vi "Banda_HMI_UART.vi"() -> ()   [LabVIEW 2026]
uses:
  <vilib>/Instr/_visa.llb/VISA Configure Serial Port (Instr).vi
panel:
  in  "VELOCIDAD BANDA":u8(knob) scale=0.0..100.0 scale format="%^#.6g"
  in  "BRAZO CLASIFICADOR":bool
  in  "MOTOR BANDA":bool
  out "Trama":bool
  in  "stop":bool
  out "CONTADOR PIEZAS":u16
  out "SENSOR DE PRESENCIA":bool
  out "TEMPERATURA":u8(slide) scale=0.0..100.0
  out "SOBRECALENTAMIENTO":bool
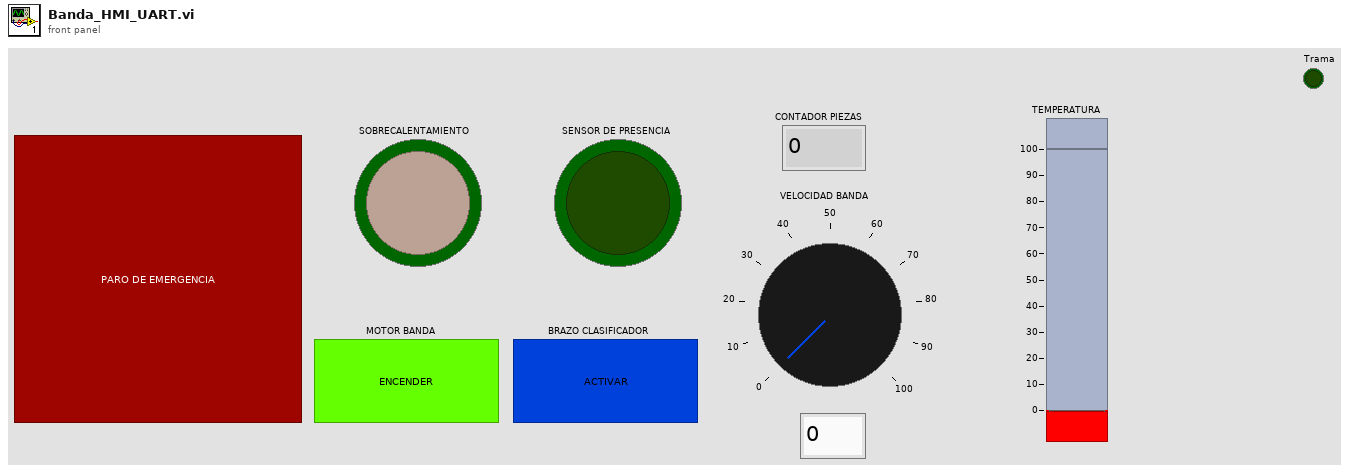
[diagram p1: front panel]
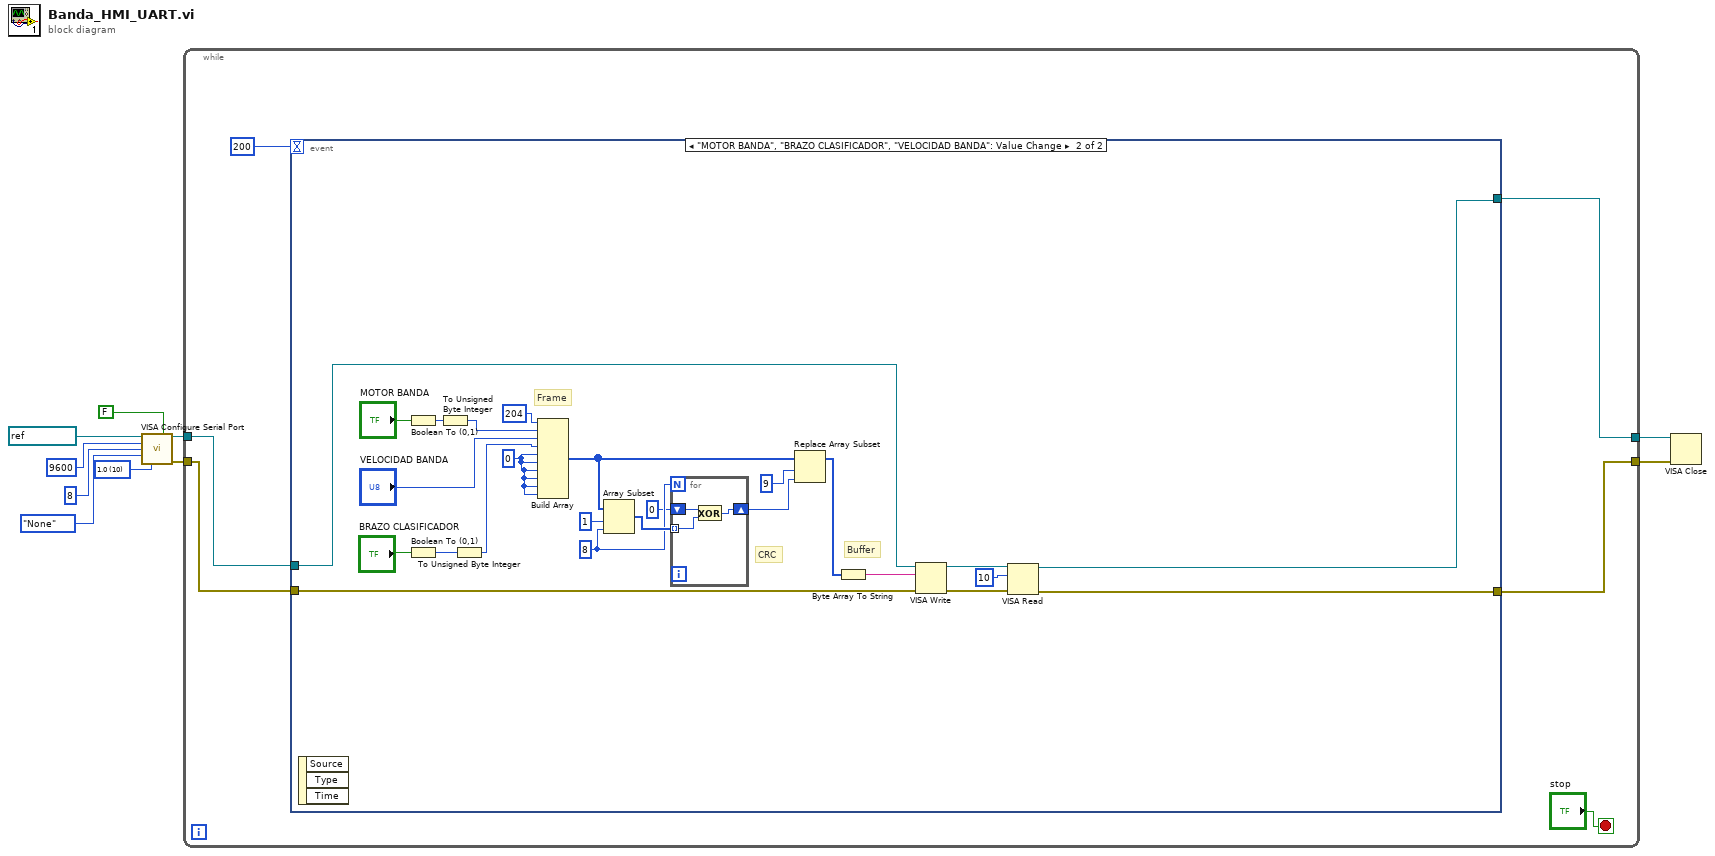
[diagram p0: block diagram]
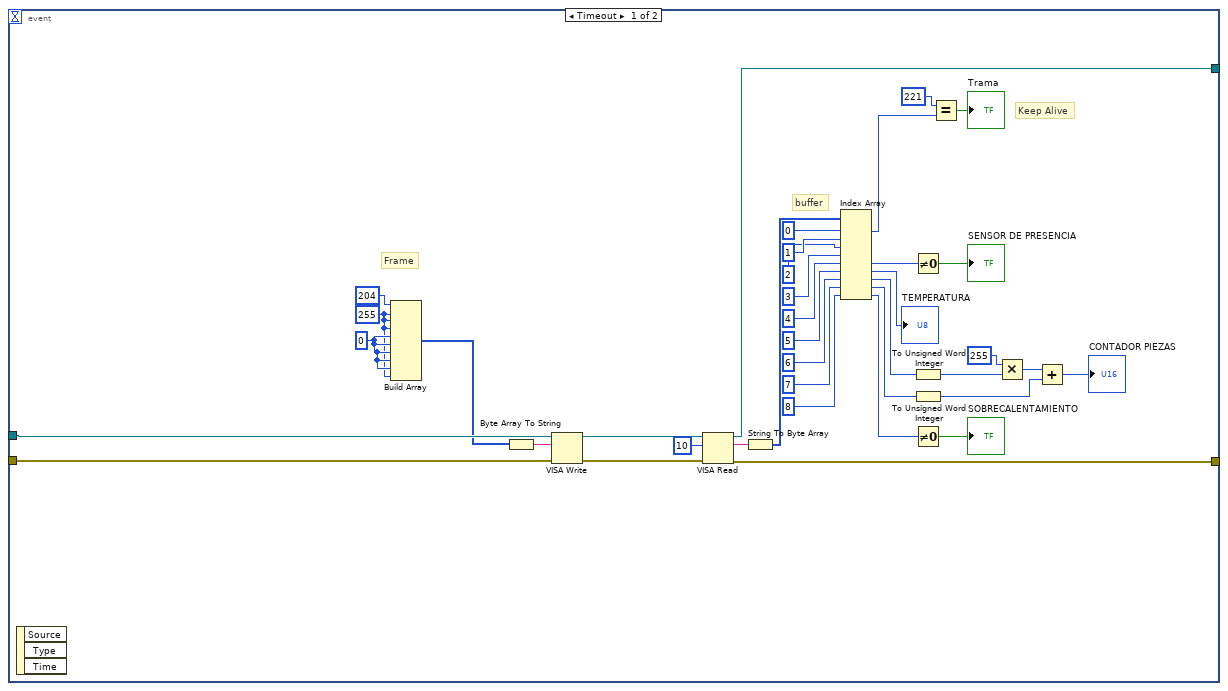
[diagram p2: hidden frame]
diagram:
  w6 = u16 10 items=["1.0"=10, "1.5"=15, "2.0"=20] ("stop bits (10: 1 bit)")
  n1 = call-poly "VISA Configure Serial Port"("VISA resource name"=refnum<visa-resource-name> "COM15", "Enable Termination\nChar (T)"=FALSE ("Enable Termination\nChar (T)"), "baud rate (9600)"=u32 9600, "data bits (8)"=u16 8, "parity (0:none)"=enum16{"None", "Odd", "Even", "Mark", "Space"}."None", "stop bits (10: 1 bit)"=w6) -> ("VISA resource name out"=w3:refnum<visa-resource-name>, "error out"=w2:errorcluster)  [unwired: 8 in]
  n2 = while {
    tunnel: w3 -> [w15]
    tunnel: [w12] -> w4
    tunnel: w2 -> [w14]
    tunnel: [w11] -> w1
    stop <- "stop" stop-if-true
    n3 = event shown="[1] \"MOTOR BANDA\", \"BRAZO CLASIFICADOR\", \"VELOCIDAD BANDA\": Value Change" {
      selector: _ -> [_ _]
      dyn-events: _ -> [_ _]
      timeout: 200 -> [_ _]
      tunnel: w15 -> [w19 w62]
      tunnel: w14 -> [w20 w61]
      tunnel: [w24 w57] -> w11
      tunnel: [w23 w58] -> w12
      event Timeout {
        w17 = u8 255 ("element")
        w52 = u8 0 ("element")
        # "Keep Alive"
        # "buffer"
        # "Frame"
        n4 = event-data() -> ()  [unwired: 1 in, 3 out]
        n5 = Build Array(u8 204 ("element"), w17, w17, w17, w52, w52, w52, w52, w52, w17) -> (w18:u8[])
        n6 = Byte Array To String(unsigned byte array=w18) -> (string=w54:string)
        n7 = VISA Write(VISA resource name=w19, write buffer=w54, error in (no error)=w20) -> (VISA resource name out=w21:refnum<visa-resource-name>, error out=w22:errorcluster)  [unwired: 1 out]
        n8 = VISA Read(VISA resource name=w21, byte count=u32 10, error in (no error)=w22) -> (VISA resource name out=w23:refnum<visa-resource-name>, read buffer=w46:string, error out=w24:errorcluster)  [unwired: 1 out]
        n9 = String To Byte Array(string=w46) -> (unsigned byte array=w49:u8[])
        n10 = Index Array(array=w49, index #1=0 ("index"), index #2=1 ("index"), index #3=2 ("index"), index #4=3 ("index"), index #5=4 ("index"), index #6=5 ("index"), index #7=6 ("index"), index #8=7 ("index"), index #9=8 ("index")) -> (element #1=w47:u8, element #5=w45:u8, element #6=→"TEMPERATURA":u8, element #7=w39:u8, element #8=w40:u8, element #9=w42:u8)  [unwired: 3 out]
        n11 = Not Equal To 0?(x=w45) -> (x != 0?=→"SENSOR DE PRESENCIA":bool)
        n12 = To Unsigned Word Integer(number=w39) -> (unsigned 16bit integer=w50:u16)
        n13 = To Unsigned Word Integer(number=w40) -> (unsigned 16bit integer=w51:u16)
        n14 = Not Equal To 0?(x=w42) -> (x != 0?=→"SOBRECALENTAMIENTO":bool)
        n15 = Equal?(x=u8 221, y=w47) -> (x = y?=→"Trama":bool)
        n16 = Multiply(x=u16 255, y=w50) -> (x*y=w37:u16)
        n17 = Add(x=w37, y=w51) -> (x+y=→"CONTADOR PIEZAS":u16)
      }
      event "MOTOR BANDA", "BRAZO CLASIFICADOR", "VELOCIDAD BANDA": Value Change {
        w75 = 8 ("length")
        w71 = u8 0 ("element")
        # "Frame"
        # "Buffer"
        # "CRC"
        n18 = event-data() -> ()  [unwired: 1 in, 3 out]
        n19 = Boolean To (0,1)(Boolean="MOTOR BANDA") -> (0, 1=w66:i16)
        n20 = Boolean To (0,1)(Boolean="BRAZO CLASIFICADOR") -> (0, 1=w69:i16)
        n21 = To Unsigned Byte Integer(number=w66) -> (unsigned 8bit integer=w64:u8)
        n22 = To Unsigned Byte Integer(number=w69) -> (unsigned 8bit integer=w65:u8)
        n23 = Build Array(u8 204 ("element"), w64, "VELOCIDAD BANDA", w65, w71, w71, w71, w71, w71, w71) -> (w78:u8[])
        n24 = Array Subset(array=w78, index=1, length=w75) -> (w77:u8[])
        n25 = for {
          N: w75 -> [_]
          shift-right: [w82] -> w55
          shift-left: 0 -> [w81]
          tunnel: w77 -> [w80] mode=indexing
          n26 = Exclusive Or(1:w80, 2:w81) -> (0:w82:i32)
        }
        n27 = Replace Array Subset(array=w78, new element=w55, index=9) -> (w79:u8[])
        n28 = Byte Array To String(unsigned byte array=w79) -> (string=w63:string)
        n29 = VISA Write(VISA resource name=w62, write buffer=w63, error in (no error)=w61) -> (VISA resource name out=w59:refnum<visa-resource-name>, error out=w60:errorcluster)  [unwired: 1 out]
        n30 = VISA Read(VISA resource name=w59, byte count=u32 10, error in (no error)=w60) -> (VISA resource name out=w58:refnum<visa-resource-name>, error out=w57:errorcluster)  [unwired: 2 out]
      }
    }
  }
  n31 = VISA Close(VISA resource name=w4, error in (no error)=w1) -> ()  [unwired: 1 out]
